vi "Handle REGISTERED.vi"(0 "WAMP Client in":refnum<class "WAMP Client.lvclass">, 5 "Message Loop Shift Register Data":T1, 7 "WAMP Message":T16 {"Message Codes" items=["HELLO"=1, "WELCOME"=2, "ABORT"=3, "GOODBYE"=6, "ERROR"=8, "PUBLISH"=16, "PUBLISHED"=17, "SUBSCRIBE"=32, "SUBSCRIBED"=33, "UNSUBSCRIBE"=34, "UNSUBSCRIBED"=35, "EVENT"=36, "CALL"=48, "RESULT"=59, "REGISTER"=64, "REGISTERED"=65, "UNREGISTER"=66, "UNREGISTERED"=67, "INVOCATION"=68, "YIELD"=70]}, 11 "error in (no error)":errorcluster) -> (4 "WAMP Client out":refnum<class "WAMP Client.lvclass">, 6 "output cluster":T1, 15 "error out":errorcluster)   [LabVIEW 2020, in "wamplv.lvlib" / "WAMP Client.lvclass"]
uses:
  WAMP Client.lvclass
  TypeDef/WAMP Received Message.ctl
  TypeDef/WAMP Message Codes.ctl
  TypeDef/Message Loop Data.ctl
  TypeDef/REGISTER Request Data.ctl
  TypeDef/Success or error.ctl
  API/TypeDefs/Combined error.ctl
  API/TypeDefs/WAMP error.ctl
  TypeDef/Publish Requests Map.ctl
  TypeDef/PUBLISH Request Data.ctl
  TypeDef/PUBLISH result.ctl
  TypeDef/Endpoint Data.ctl
  TypeDef/CALL Request Map.ctl
  Private/TypeDefs/CALL request (JSON).ctl
  API/TypeDefs/RESULT payload (JSON).ctl
  TypeDef/SUBSCRIBE Requests Map.ctl
  TypeDef/SUBSCRIBE Request Data.ctl
  TypeDef/Subscribe Result.ctl
  TypeDef/EVENT payload.ctl
  TypeDef/Subscriptions Map.ctl
  TypeDef/Subscription Details.ctl
  TypeDef/Unsubscribe Requests Map.ctl
  TypeDef/UNSUBSCRIBE Request Data.ctl
  TypeDef/UNSUBSCRIBE Result.ctl
  TypeDef/Unregister requests map.ctl
  TypeDef/Unregister request.ctl
  5b37c1c1-72ae-4897-b342-0d2a0337a4d4.vi
  WAMP Client.lvclass/WAMP Client.ctl
  wamplv.lvlib
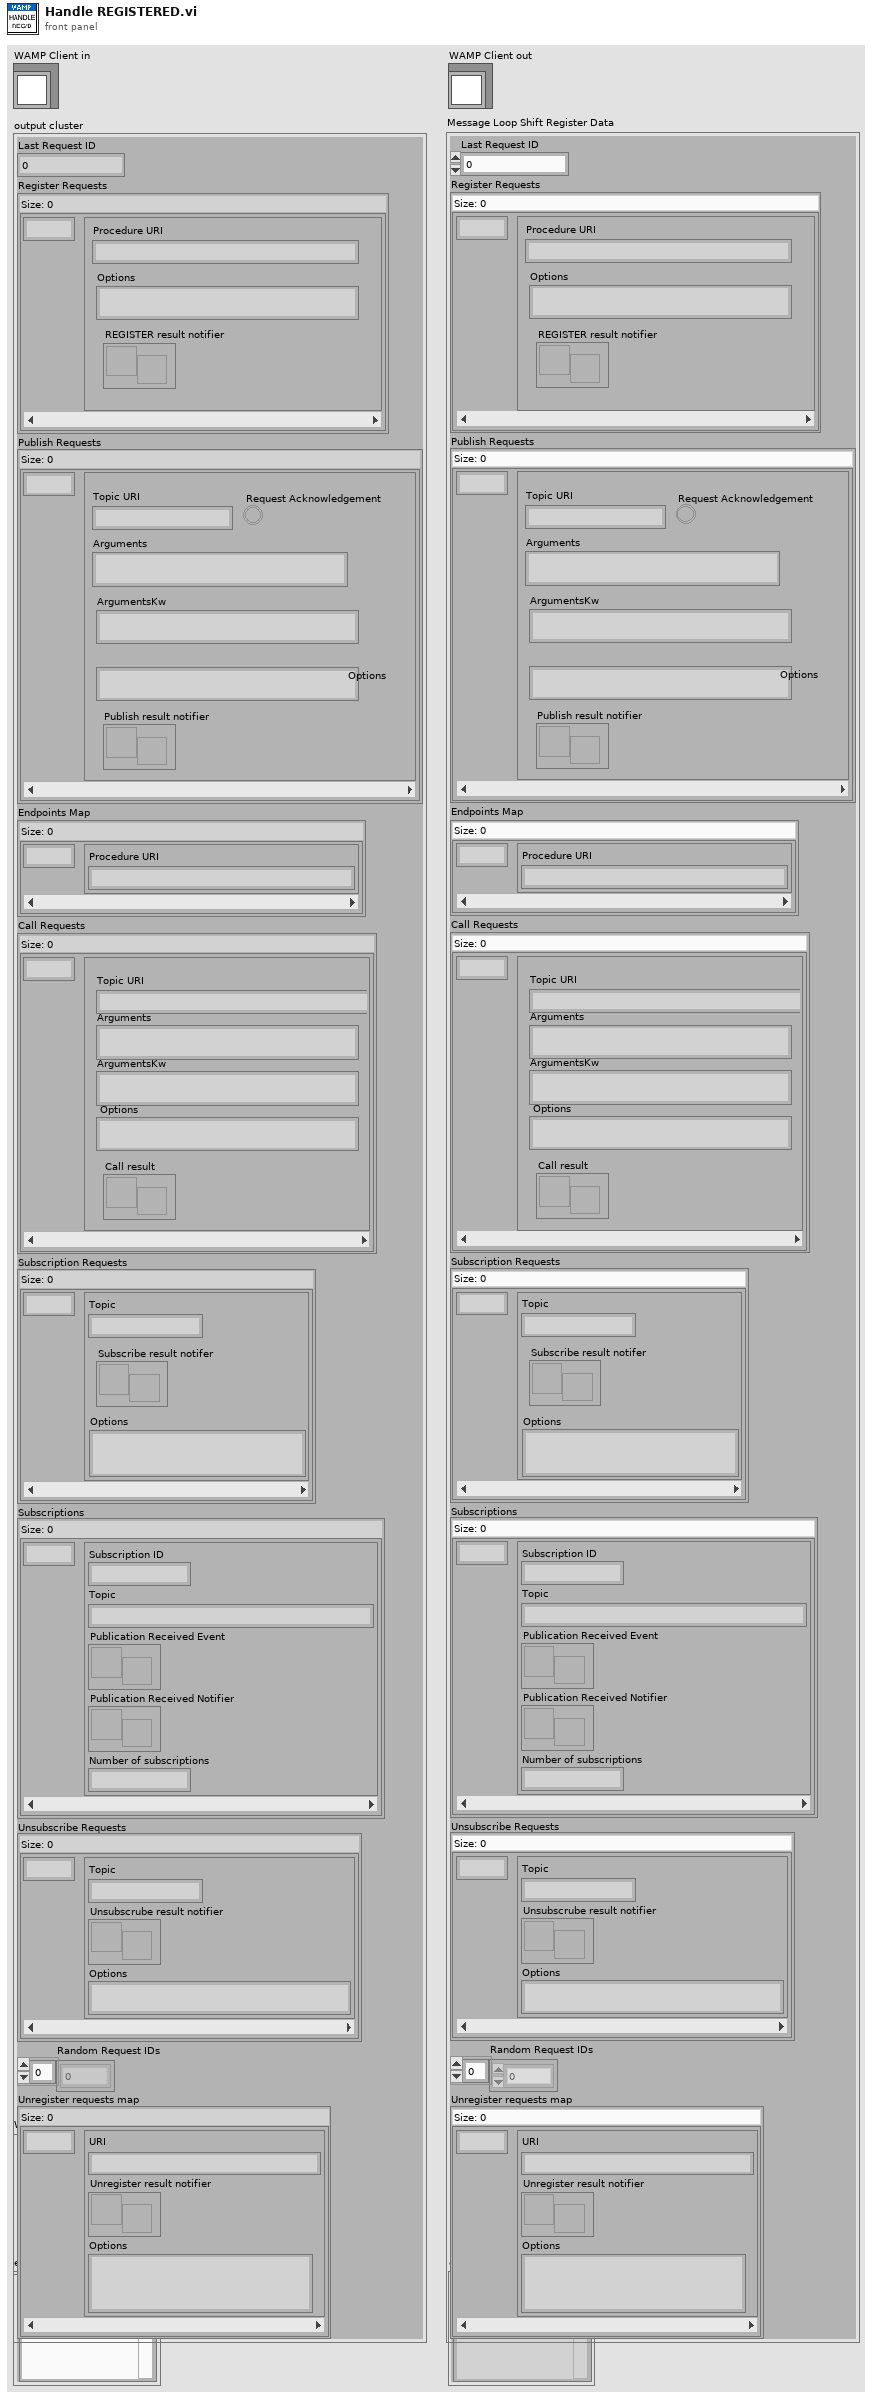
[diagram p1: front panel]
types:
  T1 = typedef "wamplv.lvlib/WAMP Client.lvclass/Message Loop Data.ctl" = cluster{"Last Request ID":u64, "Register Requests":map{u64, T2}, "Publish Requests":T3, "Endpoints Map":map{u64, T5}, "Call Requests":T6, "Subscription Requests":T8, "Subscriptions":T10, "Unsubscribe Requests":T12, "Random Request IDs":u64[], "Unregister requests map":T14}
  T2 = typedef "wamplv.lvlib/WAMP Client.lvclass/REGISTER Request Data.ctl" = cluster{"Procedure URI":string, "Options":string, "REGISTER result notifier":refnum<notifier>}
  T3 = typedef "wamplv.lvlib/WAMP Client.lvclass/Publish Requests Map.ctl" = map{u64, T4}
  T4 = typedef "wamplv.lvlib/WAMP Client.lvclass/PUBLISH Request Data.ctl" = cluster{"Topic URI":string, "Arguments":string, "ArgumentsKw":string, "Request Acknowledgement":bool, "Options":string, "Publish result notifier":refnum<notifier>}
  T5 = typedef "wamplv.lvlib/WAMP Client.lvclass/Endpoint Data.ctl" = cluster{"Procedure URI":string}
  T6 = typedef "wamplv.lvlib/WAMP Client.lvclass/CALL Request Map.ctl" = map{u64, T7}
  T7 = typedef "wamplv.lvlib/CALL request (JSON).ctl" = cluster{"Topic URI":string, "Arguments":string, "ArgumentsKw":string, "Options":string, "Call result":refnum<notifier>}
  T8 = typedef "wamplv.lvlib/WAMP Client.lvclass/SUBSCRIBE Requests Map.ctl" = map{u64, T9}
  T9 = typedef "wamplv.lvlib/WAMP Client.lvclass/SUBSCRIBE Request Data.ctl" = cluster{"Topic":string, "Subscribe result notifer":refnum<notifier>, "Options":string}
  T10 = typedef "wamplv.lvlib/WAMP Client.lvclass/Subscriptions Map.ctl" = map{u64, T11}
  T11 = typedef "wamplv.lvlib/WAMP Client.lvclass/Subscription Details.ctl" = cluster{"Subscription ID":u64, "Topic":string, "Publication Received Event":refnum<user-event>, "Publication Received Notifier":refnum<notifier>, "Number of subscriptions":u64}
  T12 = typedef "wamplv.lvlib/WAMP Client.lvclass/Unsubscribe Requests Map.ctl" = map{u64, T13}
  T13 = typedef "wamplv.lvlib/WAMP Client.lvclass/UNSUBSCRIBE Request Data.ctl" = cluster{"Topic":string, "Unsubscrube result notifier":refnum<notifier>, "Options":string}
  T14 = typedef "wamplv.lvlib/WAMP Client.lvclass/Unregister requests map.ctl" = map{u64, T15}
  T15 = typedef "wamplv.lvlib/WAMP Client.lvclass/Unregister request.ctl" = cluster{"URI":string, "Unregister result notifier":refnum<notifier>, "Options":string}
  T16 = typedef "wamplv.lvlib/WAMP Client.lvclass/WAMP Received Message.ctl" = cluster{"Message Codes":T17, "Message JSON":string[], "Bytes":u8[]}
  T17 = typedef "wamplv.lvlib/WAMP Client.lvclass/WAMP Message Codes.ctl" = u16
  T18 = typedef "wamplv.lvlib/WAMP Client.lvclass/Success or error.ctl" = cluster{"Success?":bool, "URI":string, "Combined Error":T19}
  T19 = typedef "wamplv.lvlib/WAMP Client.lvclass/Combined error.ctl" = cluster{"Error?":bool, "WAMP Error":T20, "Error":errorcluster}
  T20 = typedef "wamplv.lvlib/WAMP Client.lvclass/WAMP error.ctl" = cluster{"Details":string, "ArgumentKw Payload":string, "Error?":bool, "Error URI":string, "Arguments Payload":string}
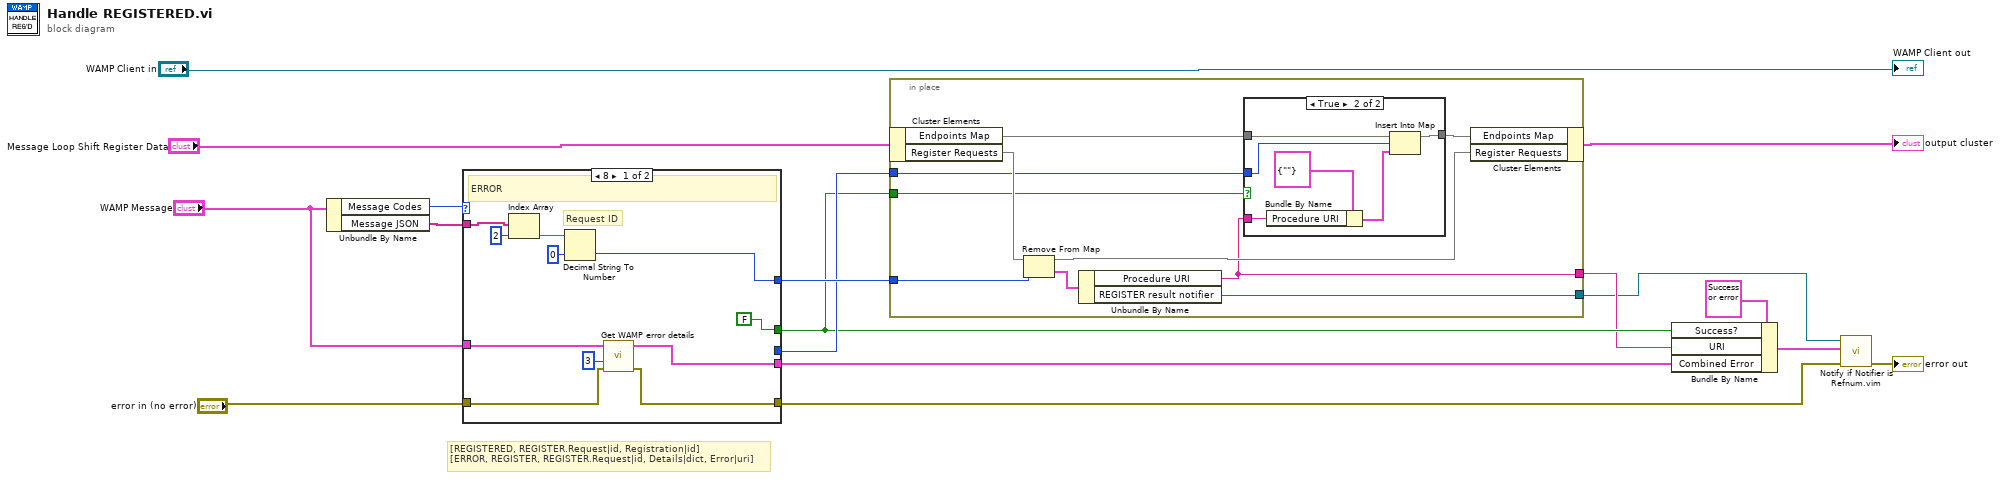
[diagram p0: block diagram]
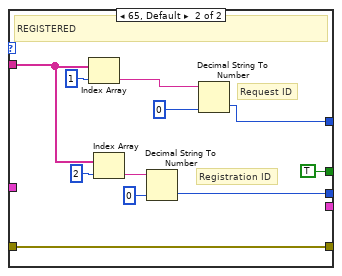
[diagram p3: hidden frame]
diagram:
  # "[REGISTERED, REGISTER.Request|id, Registration|id]\n[ERROR, REGISTER, REGISTER.Request|id, Details|dict, Error|uri]"
  n1 = Unbundle By Name("WAMP Message") -> ("Message Codes"=w16:T17, "Message JSON"=w15:string[])
  n2 = case shown="8" w16 {
    tunnel: w15 -> [w24 w32]
    tunnel: [w25 w31] -> w6
    tunnel: "error in (no error)" -> [w18 w30]
    tunnel: [w19 w30] -> w9
    tunnel: [FALSE ("Success?") TRUE ("Success?")] -> w4
    tunnel: [_ w29] -> w5
    tunnel: "WAMP Message" -> [w22 _]
    tunnel: [w20 _] -> w11
    frame 8 {
      # "Request ID"
      # "ERROR"
      n3 = Index Array(array=w24, index=2) -> (element=w27:string)
      n4 = Decimal String To Number(string=w27, default (0L)=u32 0) -> (number=w25:u32)  [unwired: 1 in, 1 out]
      n5 = call "Get WAMP error details.vi"("error in (no error)"=w18, "Details Index"=u32 3, "WAMP Message"=w22) -> ("error out"=w19:errorcluster, "Combined Error"=w20:T19)  [unwired: 6 in, 1 out]
    }
    frame 65, Default {
      # "Request ID"
      # "Registration ID"
      # "REGISTERED"
      n6 = Index Array(array=w32, index=1) -> (element=w35:string)
      n7 = Index Array(array=w32, index=2) -> (element=w38:string)
      n8 = Decimal String To Number(string=w38, default (0L)=u64 0) -> (number=w29:u64)  [unwired: 1 in, 1 out]
      n9 = Decimal String To Number(string=w35, default (0L)=u64 0) -> (number=w31:u64)  [unwired: 1 in, 1 out]
    }
  }
  n10 = in-place {
    in-place-border: w6 -> [w48]
    in-place-border: w5 -> [w45]
    in-place-border: [w42] -> w2
    in-place-border: w4 -> [w40]
    in-place-border: [w41] -> w3
    n11 = in-place-cluster #1("Message Loop Shift Register Data") -> ("Endpoints Map"=w47:map{u64, T5}, "Register Requests"=w46:map{u64, T2})
    n12 = Remove From Map(10:w48, 11:w46) -> (1:w49:T2, 3:w43:map{u64, T2})  [unwired: 1 out]
    n13 = Unbundle By Name(w49) -> ("Procedure URI"=w41:string, "REGISTER result notifier"=w42:refnum<notifier>)
    n14 = case shown="True" w40 {
      tunnel: w45 -> [_ w56]
      tunnel: w47 -> [w50 w52]
      tunnel: [w50 w51] -> w44
      tunnel: w41 -> [_ w54]
      frame False {
      }
      frame True {
        n15 = Bundle By Name(cluster=T5 {"Procedure URI"=""} ("Endpoint Data"), "Procedure URI"=w54) -> (w53:T5)
        n16 = Insert Into Map(map in=w52, key=w56, value=w53) -> (map out=w51:map{u64, T5})  [unwired: 2 out]
      }
    }
    n17 = in-place-cluster #1("Endpoints Map"=w44, "Register Requests"=w43) -> (→"output cluster":T1)
  }
  n18 = Bundle By Name(cluster=T18 {"Success?"=FALSE, "URI"="", "Combined Error"={"Error?"=FALSE, "WAMP Error"={"Details"="{}", "ArgumentKw Payload"="", "Error?"=FALSE, "Error URI"="", "Arguments Payload"=""}, "Error"={"status"=FALSE, "code"=0, "source"=""}}} ("REGISTERED or ERROR payload"), "Success?"=w4, "URI"=w3, "Combined Error"=w11) -> (w10:T18)
  n19 = call "Notify if Notifier is Refnum.vim"("error in (no error)"=w9, "RESULT Payload"=w10, "Notifier in"=w2) -> ("error out"=→"error out":errorcluster)  [unwired: 8 in]
  "WAMP Client out" <- "WAMP Client in"
